vi "Get Key Name.vi"(11 "Key Name in":refnum<class "Key Name.lvclass">) -> (2 "Keyname":string, 3 "Key Name out":refnum<class "Key Name.lvclass">)   [LabVIEW 2024, in "Electronic Datasheet.lvlib" / "Key Name.lvclass"]
uses:
  Key Name.lvclass
  Key Name.lvclass/Key Name.ctl
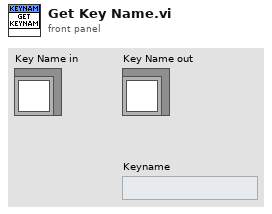
[diagram p1: front panel]
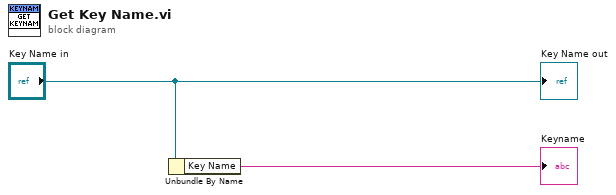
[diagram p0: block diagram]
diagram:
  n1 = Unbundle By Name("Key Name in") -> ("Key Name"=→"Keyname":string)
  "Key Name out" <- "Key Name in"
